vi "Is a valid image.vi"(0 "Image path":path, 11 "error in (no error)":errorcluster) -> (4 "dup path":path, 6 "Valid Image?":bool, 8 "Message":string, 15 "error out":errorcluster)   [LabVIEW 2013]
doc: "Version 1.0\nDeveloped by Jean-Marc Simard\nCopyright © 2010, Exaprom Inc.\nAll rights reserved.\nLicense: BSD"
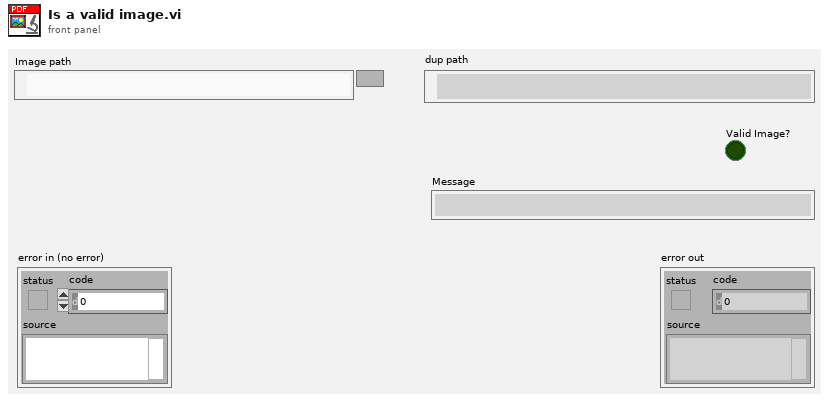
[diagram p1: front panel]
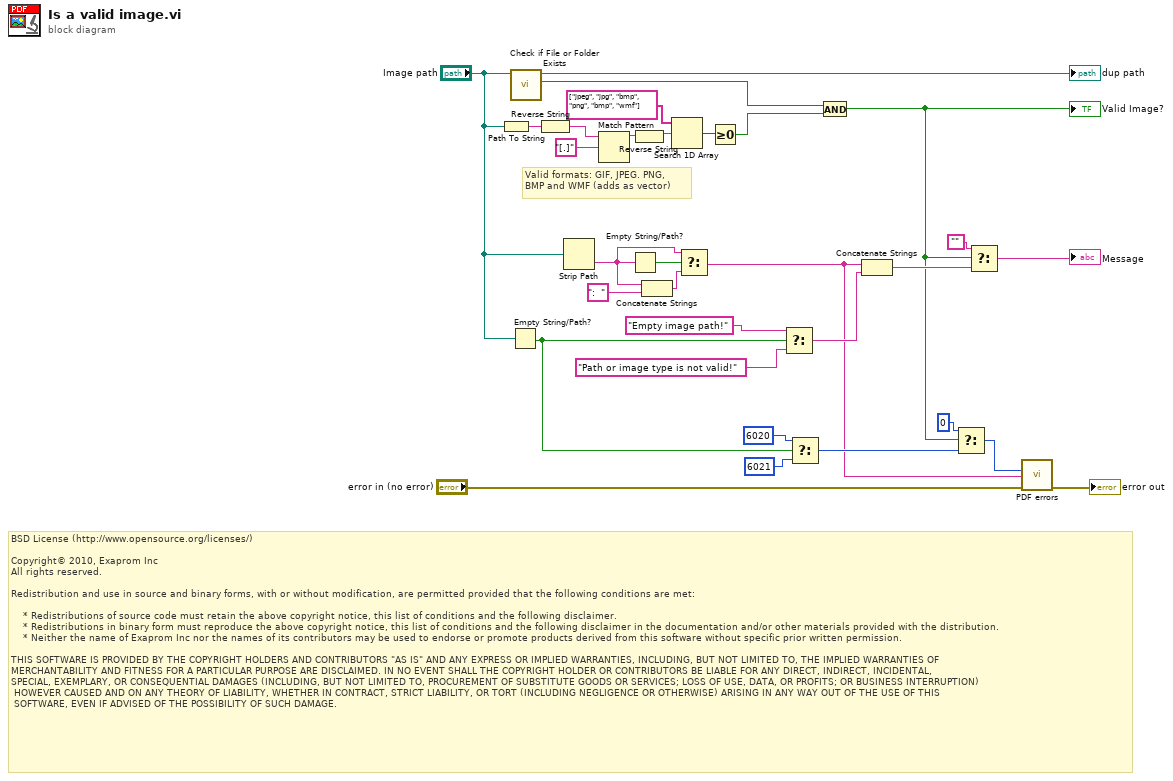
[diagram p0: block diagram]
diagram:
  # "BSD License (http://www.opensource.org/licenses/)\n\nCopyright© 2010, Exaprom Inc\nAll rights reserved.\n\nRedistribution and use in source and binary forms, with or without modification, are permitted provided that the following conditions are met:\n\n    * Redistributions of source code must retain the above copyright notice, this list of conditions and the following disclaimer.\n    * Redistributions in binary form must reproduce the above copyright notice, this list of conditions and the following disclaimer in the documentation and/or other materials provided with the distribution.\n    * Neither the name of Exaprom Inc nor the names of its contributors may be used to endorse or promote products derived from this software without specific prior written permission.\n\nTHIS SOFTWARE IS PROVIDED BY THE COPYRIGHT HOLDERS AND CONTRIBUTORS \"AS IS\" AND ANY EXPRESS OR IMPLIED WARRANTIES, INCLUDING, BUT NOT LIMITED TO, THE IMPLIED WARRANTIES OF \nMERCHANTABILITY AND FITNESS FOR A PARTICULAR PURPOSE ARE DISCLAIMED. IN NO EVENT SHALL THE COPYRIGHT HOLDER OR CONTRIBUTORS BE LIABLE FOR ANY DIRECT, INDIRECT, INCIDENTAL,\nSPECIAL, EXEMPLARY, OR CONSEQUENTIAL DAMAGES (INCLUDING, BUT NOT LIMITED TO, PROCUREMENT OF SUBSTITUTE GOODS OR SERVICES; LOSS OF USE, DATA, OR PROFITS; OR BUSINESS INTERRUPTION)\n HOWEVER CAUSED AND ON ANY THEORY OF LIABILITY, WHETHER IN CONTRACT, STRICT LIABILITY, OR TORT (INCLUDING NEGLIGENCE OR OTHERWISE) ARISING IN ANY WAY OUT OF THE USE OF THIS\n SOFTWARE, EVEN IF ADVISED OF THE POSSIBILITY OF SUCH DAMAGE."
  # "Valid formats: GIF, JPEG. PNG,\nBMP and WMF (adds as vector)"
  n1 = Path To String(path="Image path") -> (string=w26:string)
  n2 = Empty String/Path?(string/path="Image path") -> (empty?=w14:bool)
  n3 = call <vilib>:"Check if File or Folder Exists.vi"("path"="Image path") -> ("file or folder exists?"=w25:bool, "dup path"=→"dup path":path)  [unwired: 1 in, 8 out]
  n4 = Reverse String(1:w26) -> (0:w28:string)
  n5 = Strip Path(path="Image path") -> (name=w3:string)  [unwired: 1 out]
  n6 = Match Pattern(string=w28, regular expression="[.]") -> (before substring=w30:string)  [unwired: 4 out]
  n7 = Empty String/Path?(string/path=w3) -> (empty?=w5:bool)
  n8 = Reverse String(1:w30) -> (0:w31:string)
  n9 = Concatenate Strings(w3, ":  " ("string")) -> (w4:string)
  n10 = Search 1D Array(1D array=string[] ["jpeg", "jpg", "bmp", "png", "bmp", "wmf"], element=w31) -> (index of element=w24:i32)  [unwired: 1 out]
  n11 = Select(t=w3, s=w5, f=w4) -> (s? t:f=w1:string)
  n12 = Greater Or Equal To 0?(x=w24) -> (x >= 0?=w23:bool)
  n13 = Select(t="Empty image path!", s=w14, f="Path or image type is not valid!") -> (s? t:f=w16:string)
  n14 = Select(t=6020 ("code"), s=w14, f=6021 ("code")) -> (s? t:f=w9:i32)
  n15 = And(x=w25, y=w23) -> (x .and. y?=w11:bool)
  "Valid Image?" <- w11
  n16 = Concatenate Strings(w1, w16) -> (w21:string)
  n17 = Select(t=0 ("code"), s=w11, f=w9) -> (s? t:f=w6:i32)
  n18 = Select(t="", s=w11, f=w21) -> (s? t:f=→"Message":string)
  n19 = call "PDF errors.vi"("code"=w6, "Additionnal information"=w1, "error in (no error)"="error in (no error)") -> ("error out"=→"error out":errorcluster)  [unwired: 12 out]
